vi "testi5.vi"() -> ()   [LabVIEW 2015]
uses:
  BERTTA.dll
panel:
  out "Waveform Chart":dynamicdata(graph)
  in  "Setpoint":dbl
  out "temp Lauda":dbl
  out "return type":dbl
  out "rc":i32
  out "Lauda":dbl
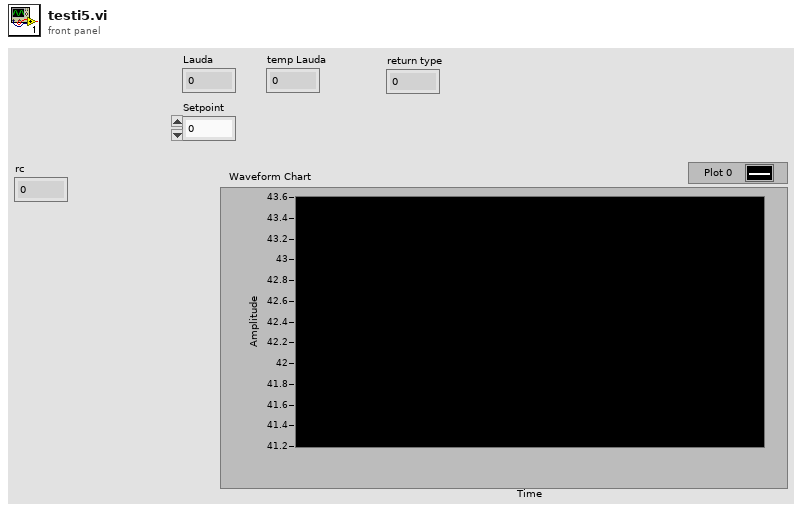
[diagram p1: front panel]
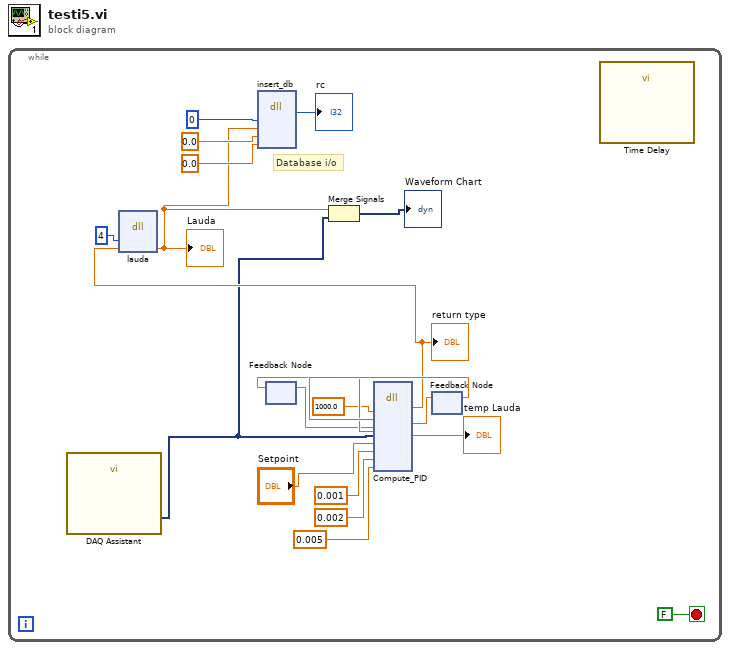
[diagram p0: block diagram]
diagram:
  n1 = while {
    stop <- FALSE stop-if-true
    # "Database i/o"
    n2 = call "DAQ Assistant"() -> ("data"=w1:dynamicdata)  [unwired: 17 in, 2 out]
    n3 = feedback #1() -> (w10:dbl)  [unwired: 1 in]
    n4 = feedback #2() -> (w13:dbl)  [unwired: 1 in]
    n5 = dll-call lib="C:/Users/xlaraser/Documents/Visual Studio 2017/Projects/Bertta/BERTTA/Debug/BERTTA.dll" fn="Compute_PID"("timeChange"=1000.0, "errSum"=w13, "lastErr"=w10, "Input"=w1, "Setpoint"="Setpoint", "kp"=0.001, "ki"=0.002, "kd"=0.005) -> ("return type"=w4:dbl, "errSum"=w14:dbl, "lastErr"=w11:dbl, "Input"=→"temp Lauda":dbl)  [unwired: 8 in, 2 out]
    "return type" <- w4
    n6 = dll-call lib="C:/Users/xlaraser/Documents/Visual Studio 2017/Projects/Bertta/BERTTA/Debug/BERTTA.dll" fn="lauda"("port"=4, "set_temp"=w4) -> ("set_temp"=w3:dbl)  [unwired: 5 in, 2 out]
    "Lauda" <- w3
    n7 = dll-call lib="C:/Users/xlaraser/Documents/Visual Studio 2017/Projects/Bertta/BERTTA/Debug/BERTTA.dll" fn="insert_db"("heidolph"=0, "lauda"=w3, "mettler1"=0.0, "mettler2"=0.0) -> ("return type"=→"rc":i32)  [unwired: 7 in, 2 out]
    n8 = feedback-in #1(w11) -> ()
    n9 = Merge Signals(w3, w1) -> (→"Waveform Chart":dynamicdata)
    n10 = feedback-in #2(w14) -> ()
    n11 = call "Time Delay"() -> ()  [unwired: 11 in, 1 out]
  }
